vi "Script_Open.vi"(1 "Script name":string, 3 "extension":string="*.rtts", 5 "error in":errorcluster, 7 "Working script":path, 9 "Saved Tree":T2[](array[typedef]), 10 "Config Cluster":T1) -> (11 "Saved tree out":T2[](array[typedef]), 13 "Working script out":path, 15 "Script name out":string, 17 "Dirty Flag":bool, 19 "error out":errorcluster)   [LabVIEW 2011]
uses:
  ScriptStepTypeDef.ctl
  Config cluster.ctl
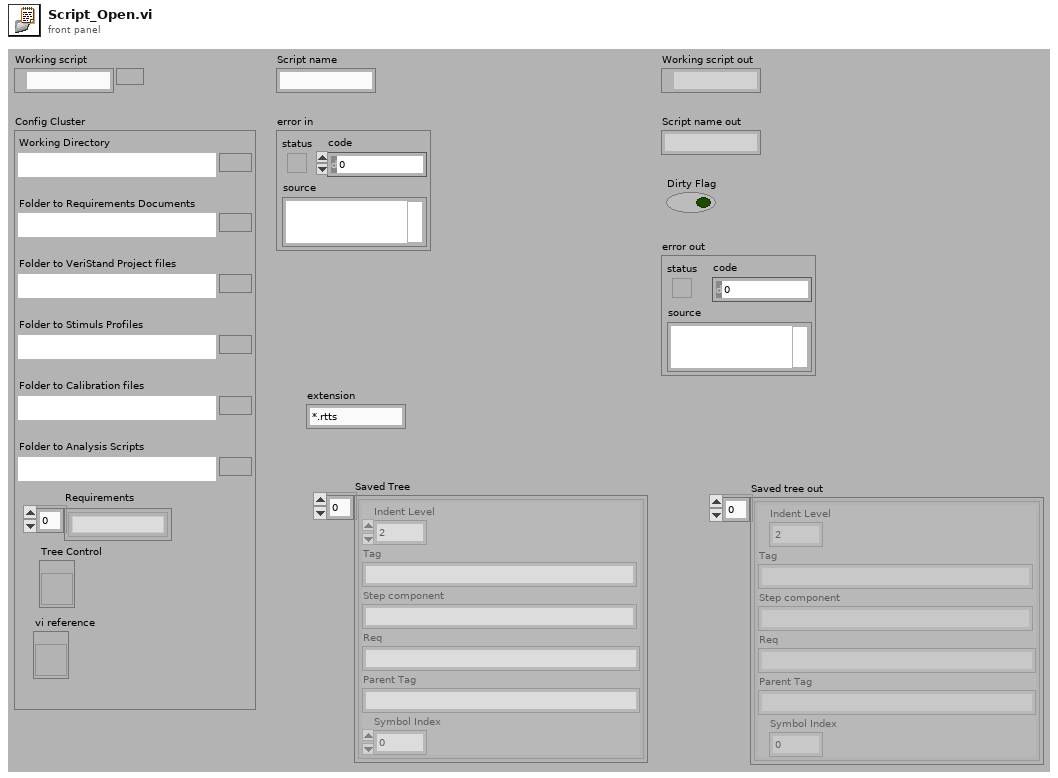
[diagram p1: front panel]
types:
  T1 = typedef "Config cluster.ctl" = cluster{"Working Directory":path, "Folder to Requirements Documents":path, "Folder to VeriStand Project files":path, "Folder to Stimuls Profiles":path, "Folder to Calibration files":path, "Folder to Analysis Scripts":path, "Requirements":string[], "Tree Control":refnum<vi>, "vi reference":refnum<vi>}
  T2 = typedef "ScriptStepTypeDef.ctl" = cluster{"Indent Level":i32, "Tag":string, "Step component":string, "Req":string, "Parent Tag":string, "Symbol Index":i32}
  T3 = enum16{"open", "replace", "create", "open or create", "replace or create", "replace or create with confirmation"}
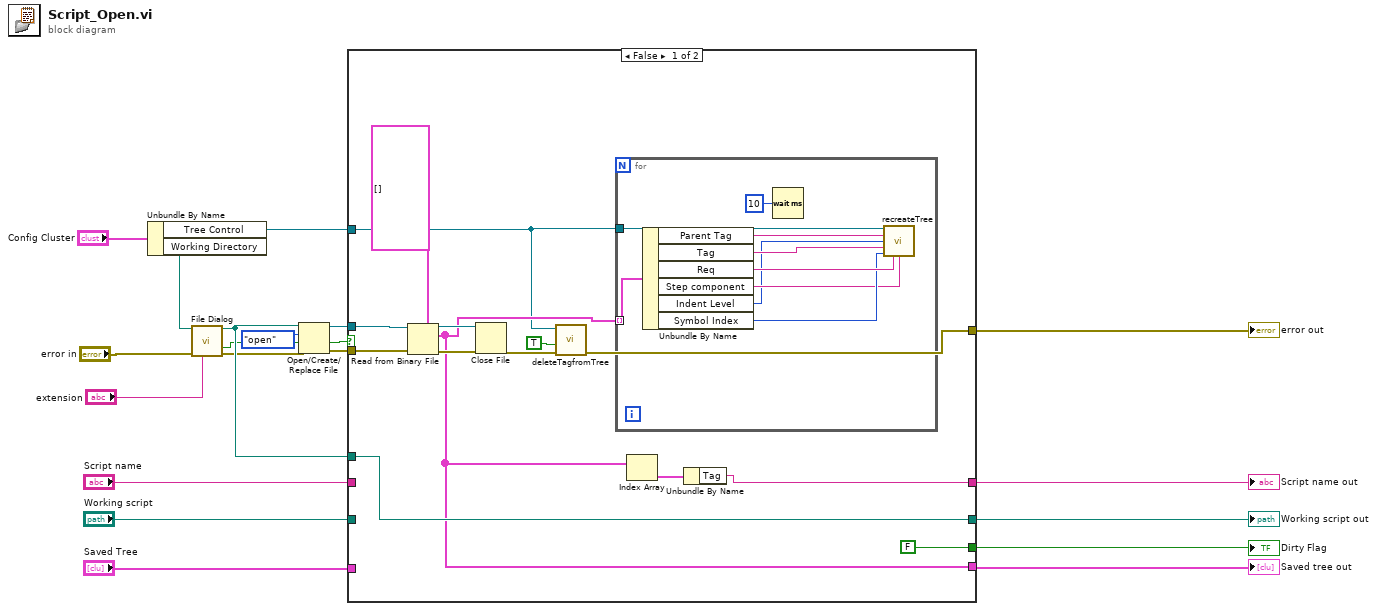
[diagram p0: block diagram]
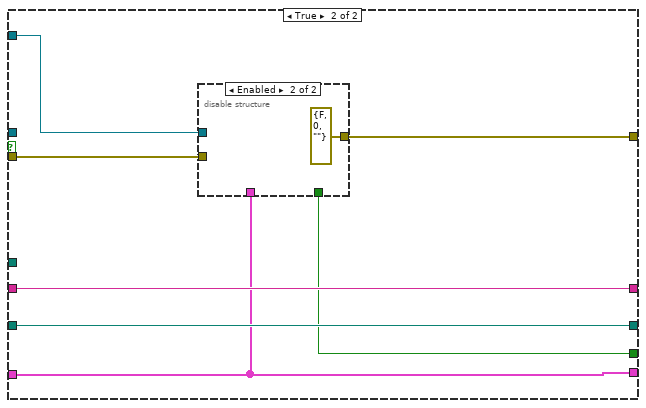
[diagram p2: hidden frame]
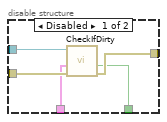
[diagram p3: hidden frame]
diagram:
  n1 = Unbundle By Name("Config Cluster") -> ("Tree Control"=w2:refnum<vi>, "Working Directory"=w12:path)
  n2 = call "File Dialog"("start path"=w12, "error in"="error in", "pattern (all files)"="extension") -> ("selected path"=w16:path, "cancelled"=w1:bool, "error out"=w9:errorcluster)  [unwired: 9 in, 1 out]
  n3 = Open/Create/Replace File(file path (use dialog)=w16, error in=w9, operation (0:open)=T3."open") -> (refnum out=w5:refnum<file>, error out=w4:errorcluster)  [unwired: 3 in, 1 out]
  n4 = case shown="False" w1 {
    tunnel: w4 -> [w33 w47]
    tunnel: w5 -> [w32 _]
    tunnel: [w26 w46] -> w6
    tunnel: "Script name" -> [_ w49]
    tunnel: [w24 w49] -> w8
    tunnel: "Working script" -> [_ w48]
    tunnel: [w23 w48] -> w15
    tunnel: w16 -> [w23 _]
    tunnel: [w22 w45] -> w17
    tunnel: "Saved Tree" -> [_ w45]
    tunnel: [FALSE w44] -> w19
    tunnel: w2 -> [w20 w43]
    frame False {
      n5 = Read from Binary File(5:T2[] [] ("Step Seq"), 8:w33, 11:w32) -> (0:w30:errorcluster, 2:w22:T2[], 3:w29:refnum<file>)  [unwired: 3 in, 1 out]
      n6 = Close File(refnum=w29, error in=w30) -> (error out=w27:errorcluster)  [unwired: 1 out]
      n7 = call "deleteTagfromTree.vi"("error in (no error)"=w27, "Delete Children?"=TRUE, "Tree Ref"=w20) -> ("error out"=w26:errorcluster)  [unwired: 7 in, 1 out]
      n8 = for {
        tunnel: w22 -> [w41] mode=indexing
        tunnel: w20 -> [w42]
        n9 = Unbundle By Name(w41) -> ("Parent Tag"=w34:string, "Tag"=w39:string, "Req"=w40:string, "Step component"=w36:string, "Indent Level"=w35:i32, "Symbol Index"=w38:i32)
        n10 = Wait (ms)(milliseconds to wait=u32 10) -> ()  [unwired: 1 out]
        n11 = call "recreateTree.vi"("Tree ref"=w42, "parent tag"=w34, "Active Item:Indent Level"=w35, "new tag"=w39, "Symbol"=w38, "Req"=w40, "Element Name"=w36) -> ()  [unwired: 9 in]
      }
      n12 = Index Array(array=w22) -> (element=w25:T2)  [unwired: 1 in]
      n13 = Unbundle By Name(w25) -> ("Tag"=w24:string)
    }
    frame True {
      n14 = disable-structure shown="Enabled" {
        disable-tunnel: w47 -> [w54 _]
        disable-tunnel: [w53 errorcluster {"status"=FALSE, "code"=0, "source"=""} ("error out")] -> w46
        disable-tunnel: w45 -> [w52 _]
        disable-tunnel: [w51 _] -> w44
        disable-tunnel: w43 -> [w50 _]
        frame Disabled {
          n15 = call "CheckIfDirty.vi"("error in"=w54, "Saved Tree"=w52, "Tree Control"=w50) -> ("error out"=w53:errorcluster, "Dirty Flag"=w51:bool)  [unwired: 6 in, 1 out]
        }
        frame Enabled {
        }
      }
    }
  }
  "Dirty Flag" <- w19
  "Saved tree out" <- w17
  "Working script out" <- w15
  "Script name out" <- w8
  "error out" <- w6
